vi "uStringManipulation_DO.vi"(8 "error in (no error)":errorcluster, 10 "String in":string, 11 "addPrefix in":refnum<class "addPrefix.lvclass">) -> (0 "error out":errorcluster, 2 "String":string, 3 "addPrefix out":refnum<class "addPrefix.lvclass">)   [LabVIEW 2021, in "uFramework_pack_uStringManipulation.lvlib" / "addPrefix.lvclass"]
uses:
  addPrefix.lvclass
  addPrefix.lvclass/addPrefix.ctl
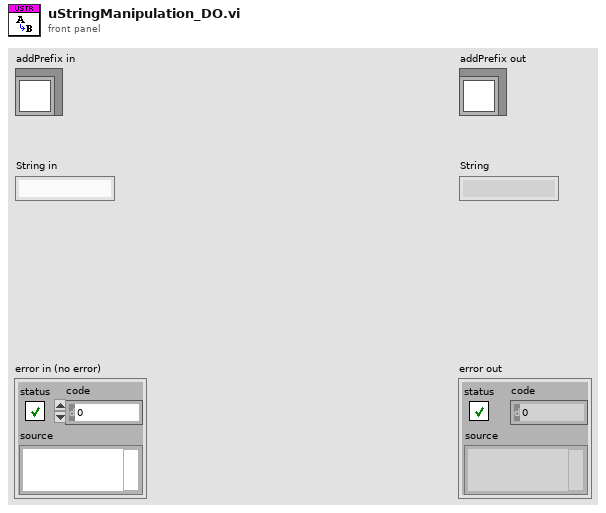
[diagram p1: front panel]
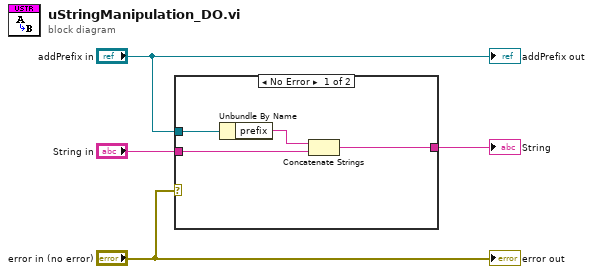
[diagram p0: block diagram]
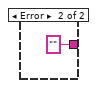
[diagram p2: hidden frame]
diagram:
  n1 = case shown="No Error" "error in (no error)" {
    tunnel: "String in" -> [w8 _]
    tunnel: [w7 ""] -> w2
    tunnel: "addPrefix in" -> [w6 _]
    frame No Error {
      n2 = Unbundle By Name(w6) -> ("prefix"=w5:string)
      n3 = Concatenate Strings(w5, w8) -> (w7:string)
    }
    frame Error {
    }
  }
  "String" <- w2
  "error out" <- "error in (no error)"
  "addPrefix out" <- "addPrefix in"
